vi "GetSamplingFromWaveform.vi"(11 "Waveforms":waveform(dbl)[](array[waveform])) -> (3 "sampling info":cluster{"Fs":dbl, "#s":dbl})   [LabVIEW 2016, in "DSP_lockin.lvclass"]
uses:
  DSP.lockin/DSP_lockin.lvclass
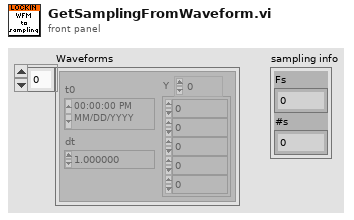
[diagram p1: front panel]
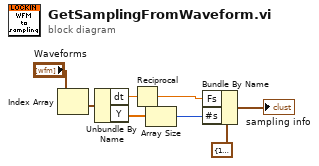
[diagram p0: block diagram]
diagram:
  n1 = Index Array(array="Waveforms") -> (element=w1:waveform(dbl))  [unwired: 1 in]
  n2 = Unbundle By Name(w1) -> ("dt"=w2:dbl, "Y"=w3:dbl[])
  n3 = Reciprocal(x=w2) -> (1/x=w7:dbl)
  n4 = Array Size(array=w3) -> (size(s)=w5:i32)
  n5 = Bundle By Name(cluster=cluster{"Fs":dbl, "#s":dbl} {"Fs"=1000.0, "#s"=1000.0} ("sampling info"), "Fs"=w7, "#s"=w5) -> (→"sampling info":cluster{"Fs":dbl, "#s":dbl})
